vi "Actor Core.vi"(8 "error in":errorcluster, 11 "SCHEMA_02 in":refnum<class "SCHEMA_02.lvclass">) -> (0 "error out":errorcluster, 3 "Actor out":refnum<class "Actor.lvclass">)   [LabVIEW 2020, in "SCHEMA_02.lvlib" / "SCHEMA_02.lvclass"]
doc: "(<B>Filename</B>: Actor Framework.lvlib:Actor.lvclass:Actor Core.vi)\n\nReceives messages to the actor, reacts to them, and initiates any error handling that may shut the actor down.\n\nDescendant classes may override this VI to append parallel tasks for the actor to complete while it handles messages. Overrides use the Call Parent Method node."
uses:
  SCHEMA_02.lvclass
  support/Actor Framework.lvlibp/1abvi3w/vi.lib/ActorFramework/Actor/Actor.lvclass
  D&C_SchemaBase/D&C_SchemaBase/D&C_SchemaBase.lvclass
panel:
  out "Source 2.pos_8":dbl caption="Source 2.Sinus" format="%-#4.3g"
  out "Source 2.pos_7":dbl caption="Source 2.Sinus" format="%-#4.3g"
  out "Source 2.pos_6":dbl caption="Source 2.Sinus" format="%-#4.3g"
  out "Source 2.pos_5":dbl caption="Source 2.Sinus" format="%-#4.3g"
  out "Source 2.pos_4":dbl caption="Source 2.Sinus" format="%-#4.3g"
  out "Source 2.pos_3":dbl caption="Source 2.Sinus" format="%-#4.3g"
  out "Source 2.pos_2":dbl caption="Source 2.Sinus" format="%-#4.3g"
  out "Source 2.pos_1":dbl caption="Source 2.Sinus" format="%-#4.3g"
  # "Source 2: les positions"
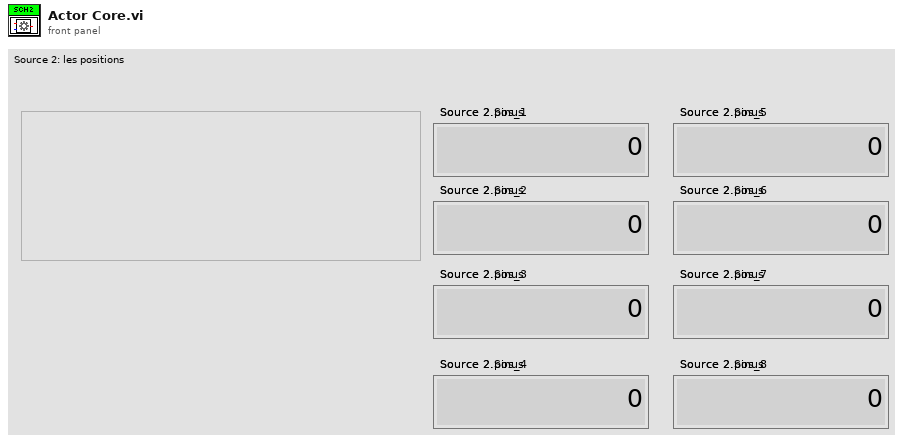
[diagram p1: front panel]
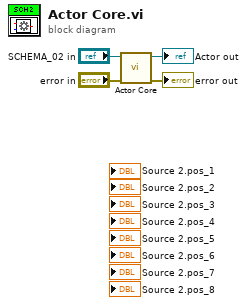
[diagram p0: block diagram]
diagram:
  n1 = call-parent "Actor Core.vi"("error in"="error in", "UI_Actor in"="SCHEMA_02 in") -> ("error out"=→"error out":errorcluster, "Actor out"=→"Actor out":refnum<class "Actor.lvclass">)  [unwired: 8 in]
